vi "PH_Waveplate-GUI_6P.constructor.vi"(0 "name":string, 2 "data in":string, 5 "error in(no error)":errorcluster) -> (14 "i ref out":refnum<vi>, 16 "data out":string, 19 "error out":errorcluster)   [LabVIEW 2014, in "PH_Waveplate-GUI_6P.lvlib"]
doc: "This class is forseen to control up to two Sixpack Axes (classes: Trinamic_Axis and Trinamic_Controller).\n\nThis class is part of the PHELIX user layer.\n\nauthor: Stefan Götte, GSI\n\nLicense Agreement for this software:\n\nCopyright (C)\nGesellschaft für Schwerionenforschung, GSI\nPlanckstr. 1\n64291 Darmstadt\nGermany\n\nContact: D.Beck@gsi.de \n\nThis program is free software; you can redistribute it and/or modify it under the terms of the \nGNU General Public License as published by the Free Software Foundation; either version 2 of \nthe license, or (at your option) any later version.\n\nThis program is distributed in the hope that it will be useful, but WITHOUT ANY WARRANTY; \nwithout even the implied warranty of MERCHANTABILITY or FITNESS FOR A PARTICULAR PURPOSE. See the GNU General License for more details (http://www.gnu.org).\n\nGesellschaft für Schwerionenforschung, GSI\nPlanckstr. 1, 64291 Darmstadt, Germany\nFor all questions and ideas contact: M.Richter@gsi.de, H.Brand@gsi.de or D.Beck@gsi.de.\nLast update: 16-JUN-2004"
uses:
  PH_Waveplate-GUI_6P.lvlib
  CSCore/CSObj/CSObj.lvlib
  PH_AxisGUI_BaseClass/PH_AxisGUI_BaseClass.lvlib
  PH_Class/PH_Class.lvlib
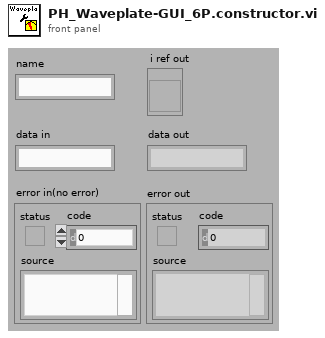
[diagram p1: front panel]
types:
  T1 = enum16{"SetAttribute", "GetAttribute", "CreateAttribute", "DestroyAttribute", "DestroyAllAtributes"}
  T2 = typedef "PH_Waveplate-GUI_6P.lvlib/PH_Waveplate-GUI_6P.i attribute.ctl" = cluster{"GUI Refs":cluster{"Meter":refnum<vi>, "Extend Limits":refnum<vi>, "Type":refnum<vi>, "Target":refnum<vi>}, "Extend Waveplate Limit":bool, "Type":T3, "Limit":dbl}
  T3 = typedef "PH_Waveplate-GUI_6P.lvlib/PH_Waveplate-GUI_6P.Type.ctl" = u16
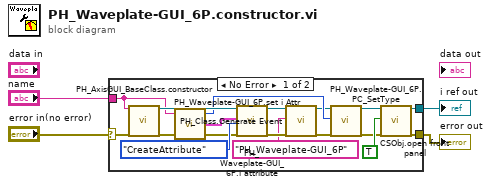
[diagram p0: block diagram]
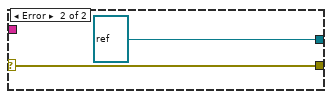
[diagram p2: hidden frame]
diagram:
  n1 = case shown="No Error" "error in(no error)" {
    selector: "error in(no error)" -> [w12 w24]
    tunnel: [w20 w24] -> w4
    tunnel: [w21 refnum<vi> refnum ("i ref out")] -> w3
    tunnel: "name" -> [w11 _]
    frame No Error {
      n2 = call "PH_AxisGUI_BaseClass.constructor.vi"("name"=w11, "error in(no error)"=w12) -> ("i ref out"=w17:refnum<vi>, "error out"=w10:errorcluster)  [unwired: 15 in, 1 out]
      n3 = call "PH_Waveplate-GUI_6P.set i Attr.vi"("error in (no error)"=w10, "Instance Name"=w11) -> ("error out"=w9:errorcluster, "i Attributes"=w8:T2, "Default Type"=w7:T3)  [unwired: 1 in]
      n4 = call "PH_Waveplate-GUI_6P.i attribute.vi"("VI Refnum"=w17, "CLASS.i attribute"=w8, "Action"=T1."CreateAttribute", "error in (no error)"=w9) -> ("VI Refnum out"=w13:refnum<vi>, "error out"=w19:errorcluster)  [unwired: 13 in, 1 out]
      n5 = call "PH_Class.Generate Event.vi"("i ref in"=w13, "Class"="PH_Waveplate-GUI_6P", "error in (no error)"=w19) -> ("i ref out"=w6:refnum<vi>, "error out"=w5:errorcluster)  [unwired: 15 in]
      n6 = call "PH_Waveplate-GUI_6P.PC_SetType.vi"("VI in"=w6, "Type"=w7, "error in"=w5) -> ("VI out"=w15:refnum<vi>, "error out"=w14:errorcluster)  [unwired: 15 in]
      n7 = call "CSObj.open front panel.vi"("i ref in"=w15, "frontPanelOpen"=TRUE ("front panel open"), "error in (no error)"=w14) -> ("i ref out"=w21:refnum<vi>, "error out"=w20:errorcluster)  [unwired: 15 in]
    }
    frame Error {
    }
  }
  "i ref out" <- w3
  "error out" <- w4
